vi "Filters.vi"() -> ()   [LabVIEW 2015]
panel:
  out "Harmonic 5":dynamicdata(graph) caption="Filtered Signal"
  out "Harmonic 4":dynamicdata(graph) caption="Filtered Signal"
  out "Harmonic 3":dynamicdata(graph) caption="Filtered Signal"
  out "Harmonic 2":dynamicdata(graph) caption="Filtered Signal"
  out "Harmonic 1":dynamicdata(graph) caption="Filtered Signal"
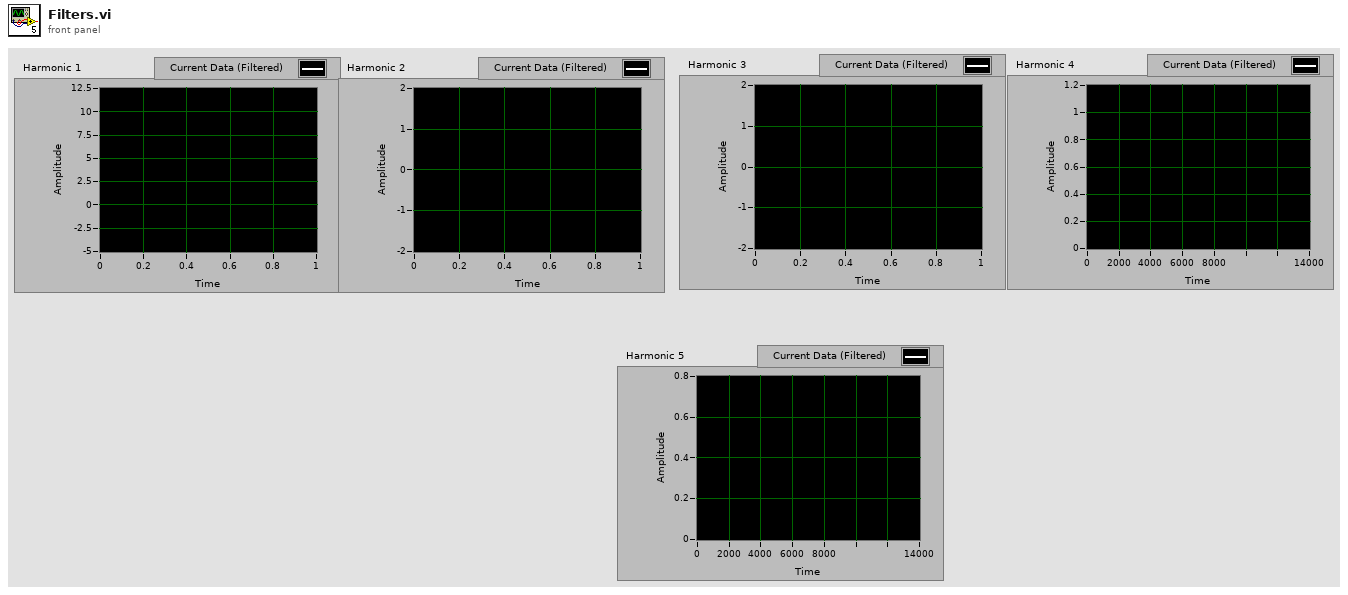
[diagram p1: front panel]
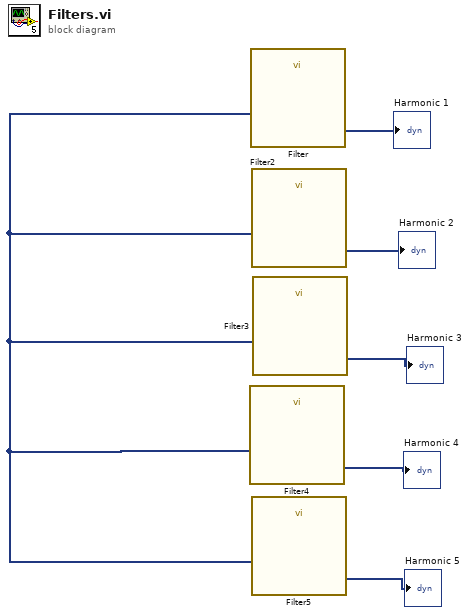
[diagram p0: block diagram]
diagram:
  n1 = call "Filter4"() -> ("Filtered Signal"=→"Harmonic 4":dynamicdata, "Signal"=w1:dynamicdata)  [unwired: 9 in, 1 out]
  n2 = call "Filter"("Signal"=w1) -> ("Filtered Signal"=→"Harmonic 1":dynamicdata)  [unwired: 9 in, 1 out]
  n3 = call "Filter2"("Signal"=w1) -> ("Filtered Signal"=→"Harmonic 2":dynamicdata)  [unwired: 9 in, 1 out]
  n4 = call "Filter5"("Signal"=w1) -> ("Filtered Signal"=→"Harmonic 5":dynamicdata)  [unwired: 9 in, 1 out]
  n5 = call "Filter3"("Signal"=w1) -> ("Filtered Signal"=→"Harmonic 3":dynamicdata)  [unwired: 9 in, 1 out]
